vi "RDS Child Receive Message.vi"(8 "error in (no error)":errorcluster, 10 "RDS Message":refnum<class "RDS Message.lvclass">, 11 "RDS Parent Actor in":refnum<class "RDS Parent Actor.lvclass">) -> (0 "error out":errorcluster, 3 "RDS Parent Actor out":refnum<class "RDS Parent Actor.lvclass">)   [LabVIEW 2015, in "RDS Abstracts.lvlib" / "RDS Parent Actor.lvlib" / "RDS Parent Actor.lvclass"]
uses:
  RDS Parent Actor.lvclass
  Libraries/RDS Framework/RDS Message Class/RDS Message.lvclass
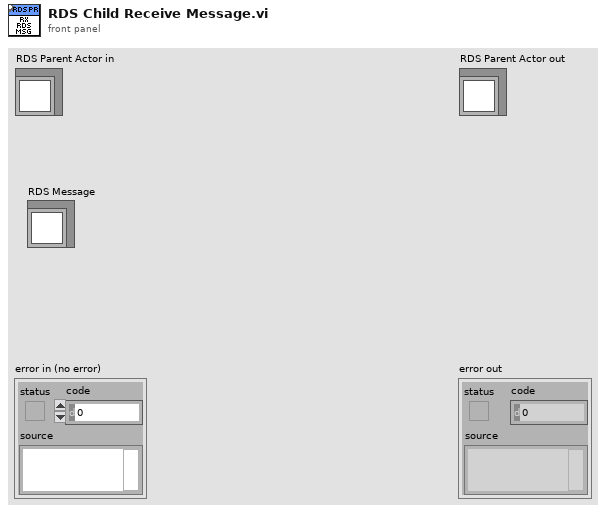
[diagram p1: front panel]
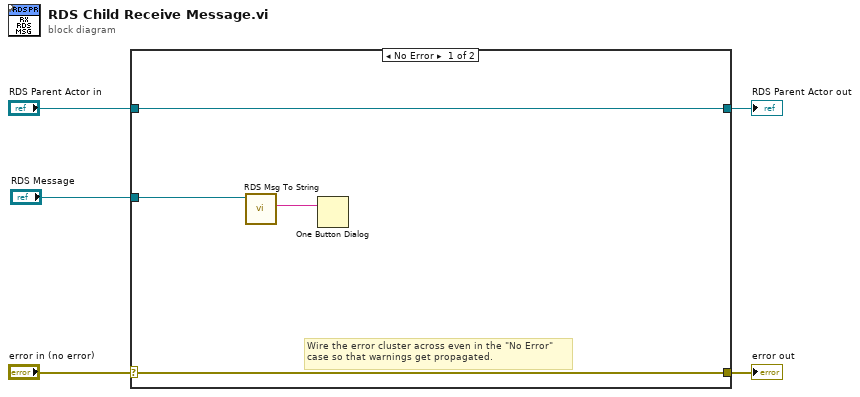
[diagram p0: block diagram]
diagram:
  n1 = case shown="No Error" "error in (no error)" {
    selector: "error in (no error)" -> [w9 w11]
    tunnel: [w9 w11] -> w4
    tunnel: [w8 w10] -> w2
    tunnel: "RDS Parent Actor in" -> [w8 w10]
    tunnel: "RDS Message" -> [w7 _]
    frame No Error {
      # "Wire the error cluster across even in the \"No Error\"\ncase so that warnings get propagated."
      n2 = call-dynamic "RDS Msg To String.vi"("RDS Message in"=w7) -> ("String"=w6:string)  [unwired: 8 in, 2 out]
      n3 = One Button Dialog(message=w6) -> ()  [unwired: 1 in, 1 out]
    }
    frame Error {
    }
  }
  "error out" <- w4
  "RDS Parent Actor out" <- w2
